vi "Main.vi"() -> ()   [LabVIEW 2015]
doc: "VI Main."
uses:
  UndoLibrary/Support VIs/DataClass/Controls/cluster_Control Value.ctl
  UndoLibrary/Support VIs/DataClass/DataObject.lvclass
  UndoLibrary/UndoClass/UndoObject.lvclass
  UndoLibrary/UndoLibrary.lvlib
panel:
  in  "City":string
  in  "Sex":enum32{"Female", "Male"}(radio)
  in  "Birthday":timestamp format="%<%x>T"
  in  "Name":string
  in  "stop":bool
  # "Run-Time Menu uses \"Edit\" User item.\n\nThe code works both in Development mode and in exe."
  # "Actual application visible front panel"
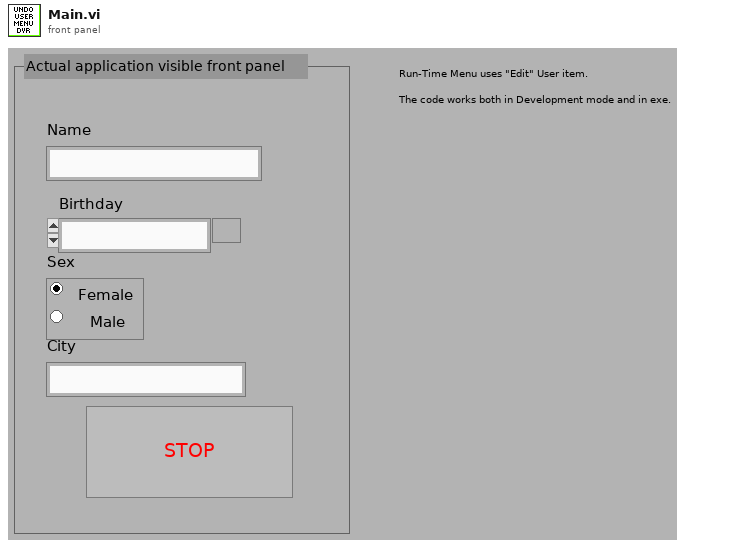
[diagram p1: front panel]
types:
  T1 = typedef "UndoLibrary.lvlib/DataObject.lvclass/cluster_Control Value.ctl" = cluster{"Index":i32, "Variant Data":variant}
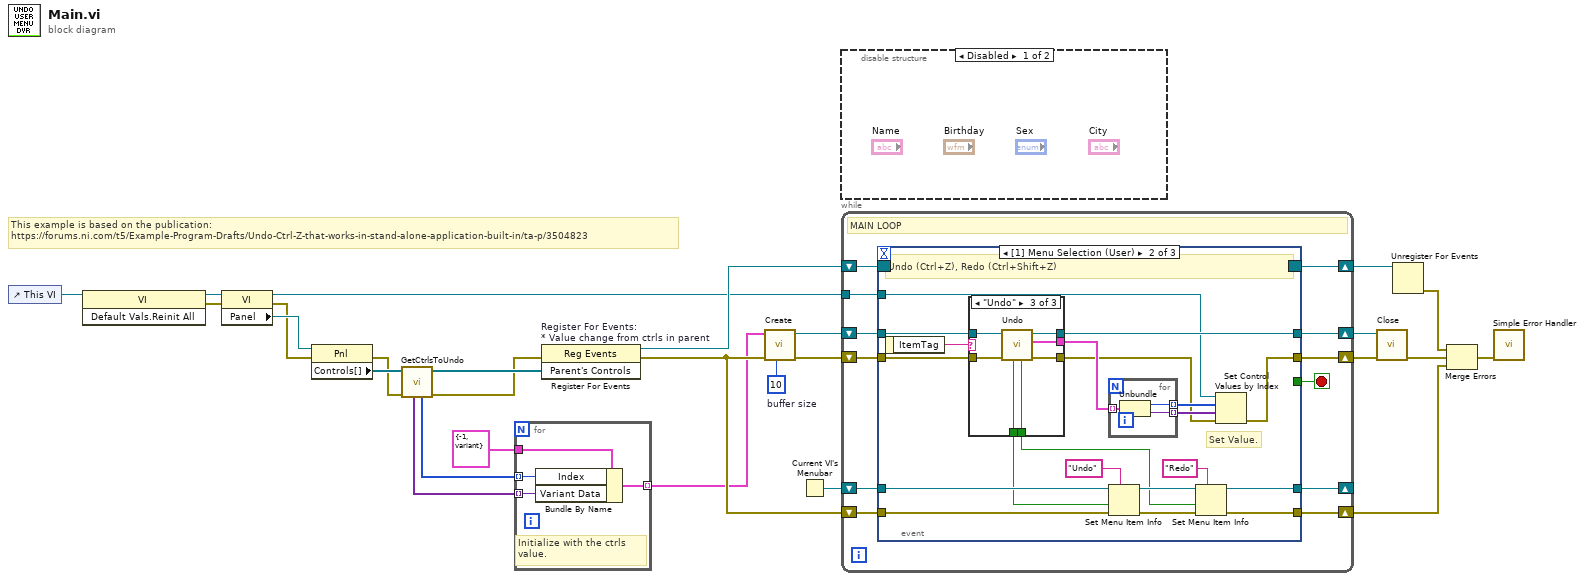
[diagram p0: block diagram]
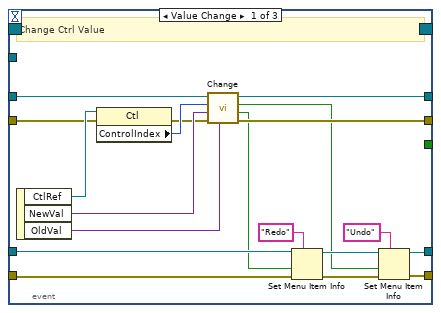
[diagram p3: hidden frame]
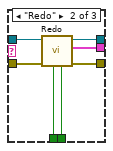
[diagram p5: hidden frame]
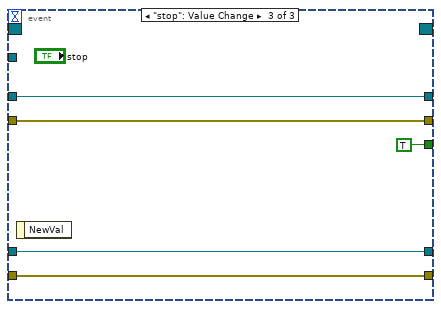
[diagram p6: hidden frame]
diagram:
  w25 = 10  # buffer size
  # "This example is based on the publication:\nhttps://forums.ni.com/t5/Example-Program-Drafts/Undo-Ctrl-Z-that-works-in-stand-alone-application-built-in/ta-p/3504823"
  n1 = control-ref of="This VI"() -> (w17:refnum<vi>)
  n2 = invoke class="VI" method="Default Vals.Reinit All"(reference=w17) -> (reference out=w16:refnum<vi>, error out=w15:errorcluster)  [unwired: 2 in, 1 out]
  n3 = property class="VI"(reference=w16, error in=w15) -> (reference out=w2:refnum<vi>, error out=w14:errorcluster, "Panel"=w27:refnum<vi>)
  n4 = property class="Pnl"(reference=w27, error in=w14) -> (error out=w12:errorcluster, "Controls[]"=w13:refnum<vi>[])  [unwired: 1 out]
  n5 = call "GetCtrlsToUndo.vi"("error in"=w12, "References\nfor Controls\non parent"=w13) -> ("error out"=w1:errorcluster, "Parent's Controls"=w11:refnum<vi>[], "Index"=w10:i32[], "Initial Values"=w9:variant[])  [unwired: 6 in]
  n6 = for {
    tunnel: [w31] -> w3 mode=indexing
    tunnel: w10 -> [w30] mode=indexing
    tunnel: w9 -> [w29] mode=indexing
    tunnel: T1 {"Index"=-1, "Variant Data"=variant} ("Control Value") -> [w28]
    # "Initialize with the ctrls\nvalue."
    n7 = Bundle By Name(cluster=w28, "Index"=w30, "Variant Data"=w29) -> (w31:T1)
  }
  n8 = register-events "Register For Events:\n* Value change from ctrls in parent"(error in=w1, w11) -> (reference out=w20:refnum<event-registration>, error out=w5:errorcluster)  [unwired: 1 in]
  n9 = call "Create.vi"("buffer size (10)"=w25, "error in (no error)"=w5, "Ctrl Val.Set All"=w3) -> ("error out"=w24:errorcluster, "UndoObject out"=w26:refnum<class "UndoObject.lvclass">)  [unwired: 7 in]
  n10 = Current VI's Menubar() -> (w6:refnum<k9>)
  n11 = disable-structure shown="Disabled" {
    frame Disabled {
    }
    frame Enabled {
    }
  }
  n12 = while {
    shift-right: [w40] -> w23
    shift-left: w26 -> [w42]
    shift-right: [w39] -> w22
    shift-left: w24 -> [w41]
    tunnel: w2 -> [w38]
    shift-right: [w36] -> w19
    shift-left: w20 -> [w37]
    shift-right: [w33] -> _
    shift-left: w6 -> [w35]
    shift-right: [w32] -> w4
    shift-left: w5 -> [w34]
    stop <- w43 stop-if-true
    # "MAIN LOOP"
    n13 = event shown="[1] Menu Selection (User)" {
      selector: w37 -> [_ _ _]
      dyn-events: [_ _ _] -> w36
      timeout: _ -> [_ _ _]
      tunnel: [w61 w78 w105] -> w40
      tunnel: w42 -> [w62 w79 w105]
      tunnel: [_ _ TRUE] -> w43
      tunnel: w41 -> [w55 w77 w104]
      tunnel: [w57 w74 w104] -> w39
      tunnel: w38 -> [_ w76 _]
      tunnel: w35 -> [w47 w68 w103]
      tunnel: w34 -> [w46 w67 w102]
      tunnel: [w49 w66 w103] -> w33
      tunnel: [w48 w65 w102] -> w32
      event Value Change {
        # "Change Ctrl Value"
        n14 = event-data() -> ("CtlRef"=w59:refnum<vi>, "NewVal"=w56:variant, "OldVal"=w60:variant)  [unwired: 1 in]
        n15 = property class="Ctl"(reference=w59, error in=w55) -> (error out=w54:errorcluster, "ControlIndex"=w58:i32)  [unwired: 1 out]
        n16 = call "Change.vi"("OldVal"=w60, "error in (no error)"=w54, "NewVal"=w56, "Control Index"=w58, "UndoObject in"=w62) -> ("error out"=w57:errorcluster, "Redo Enable"=w44:bool, "Undo Enable"=w45:bool, "UndoObject out"=w61:refnum<class "UndoObject.lvclass">)  [unwired: 3 in]
        n17 = Set Menu Item Info(7:"Redo" ("item tag"), 8:w46, 9:w44, 11:w47) -> (0:w52:errorcluster, 3:w53:refnum<k9>)  [unwired: 3 out]
        n18 = Set Menu Item Info(7:"Undo" ("item tag"), 8:w52, 9:w45, 11:w53) -> (0:w48:errorcluster, 3:w49:refnum<k9>)  [unwired: 3 out]
      }
      event Menu Selection (User) {
        # "Set Value."
        # "Undo (Ctrl+Z), Redo (Ctrl+Shift+Z)"
        n19 = event-data() -> ("ItemTag"=w73:string)  [unwired: 1 in]
        n20 = case shown="\"Undo\"" w73 {
          tunnel: [_ w88 w98] -> w82
          tunnel: w79 -> [w84 w91 w97]
          tunnel: [w84 w89 w96] -> w78
          tunnel: w77 -> [w83 w90 w95]
          tunnel: [w83 w87 w94] -> w75
          tunnel: [_ w86 w93] -> w64
          tunnel: [_ w85 w92] -> w63
          frame Default {
          }
          frame "Redo" {
            n21 = call "Redo.vi"("error in (no error)"=w90, "UndoObject in"=w91) -> ("error out"=w87:errorcluster, "Ctrl Val.Get All"=w88:T1[], "UndoObject out"=w89:refnum<class "UndoObject.lvclass">, "Redo Enable"=w85:bool, "Undo Enable"=w86:bool)  [unwired: 5 in]
          }
          frame "Undo" {
            n22 = call "Undo.vi"("error in (no error)"=w95, "UndoObject in"=w97) -> ("error out"=w94:errorcluster, "Ctrl Val.Get All"=w98:T1[], "UndoObject out"=w96:refnum<class "UndoObject.lvclass">, "Redo Enable"=w92:bool, "Undo Enable"=w93:bool)  [unwired: 5 in]
          }
        }
        n23 = for {
          tunnel: w82 -> [w101] mode=indexing
          tunnel: [w100] -> w81 mode=indexing
          tunnel: [w99] -> w80 mode=indexing
          n24 = Unbundle(w101) -> ("Index"=w100:i32, "Variant Data"=w99:variant)
        }
        n25 = Set Menu Item Info(7:"Undo" ("item tag"), 8:w67, 9:w64, 11:w68) -> (0:w71:errorcluster, 3:w72:refnum<k9>)  [unwired: 3 out]
        n26 = Set Menu Item Info(7:"Redo" ("item tag"), 8:w71, 9:w63, 11:w72) -> (0:w65:errorcluster, 3:w66:refnum<k9>)  [unwired: 3 out]
        n27 = Set Control Values by Index(0:w76, 1:w81, 2:w80, 3:w75) -> (11:w74:errorcluster)
      }
      event "stop": Value Change {
        n28 = event-data() -> ()  [unwired: 1 in, 1 out]
      }
    }
  }
  n29 = call "Close.vi"("error in (no error)"=w22, "UndoObject in"=w23) -> ("error out"=w21:errorcluster)  [unwired: 9 in]
  n30 = Unregister For Events(event registration refnum=w19) -> (error out=w18:errorcluster)  [unwired: 1 in]
  n31 = Merge Errors(w18, w21, w4) -> (w8:errorcluster)
  n32 = call <vilib>:"Simple Error Handler.vi"("error in (no error)"=w8) -> ()  [unwired: 4 in, 5 out]
